vi "QueueEvent.vi"(8 "Error In":errorcluster, 9 "Event Description":string, 10 "Event Name":string, 11 "Queue In":refnum<queue>) -> (0 "Error Out":errorcluster, 3 "Queue Out":refnum<queue>)   [LabVIEW 2014]
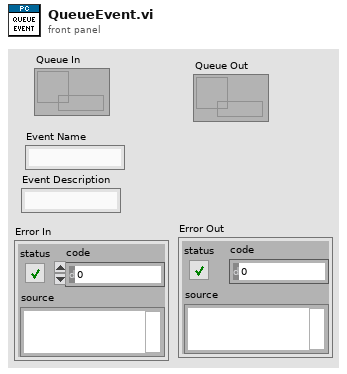
[diagram p1: front panel]
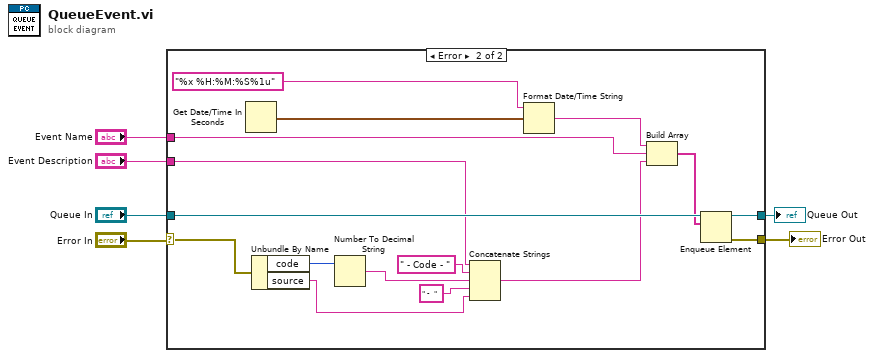
[diagram p0: block diagram]
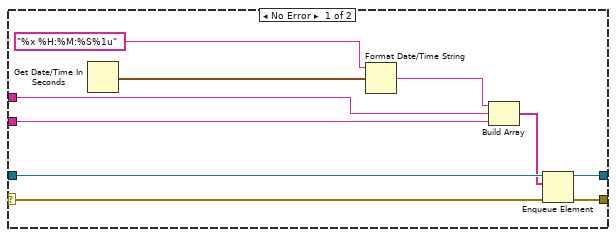
[diagram p2: hidden frame]
diagram:
  n1 = case shown="Error" "Error In" {
    selector: "Error In" -> [w11 w20]
    tunnel: [w9 w28] -> w5
    tunnel: "Queue In" -> [w10 w29]
    tunnel: "Event Name" -> [w13 w17]
    tunnel: "Event Description" -> [w12 w19]
    tunnel: [w7 w26] -> w1
    frame No Error {
      n2 = Get Date/Time In Seconds() -> (seconds since 1Jan1904=w16:timestamp)
      n3 = Format Date/Time String(time format string (%c)="%x %H:%M:%S%1u", seconds (now)=w16) -> (date/time string=w14:string)  [unwired: 1 in]
      n4 = Build Array(w14, w13, w12) -> (w8:string[])
      n5 = Enqueue Element(queue=w10, element=w8, error in (no error)=w11) -> (queue out=w7:refnum<queue>, error out=w9:errorcluster)  [unwired: 1 in, 1 out]
    }
    frame Error {
      n6 = Get Date/Time In Seconds() -> (seconds since 1Jan1904=w32:timestamp)
      n7 = Unbundle By Name(w20) -> ("code"=w25:i32, "source"=w21:string)
      n8 = Number To Decimal String(number=w25) -> (decimal integer string=w23:string)  [unwired: 1 in]
      n9 = Concatenate Strings(w19, " - Code - " ("Event Name"), w23, " -  " ("Event Name"), w21) -> (w18:string)
      n10 = Format Date/Time String(time format string (%c)="%x %H:%M:%S%1u", seconds (now)=w32) -> (date/time string=w30:string)  [unwired: 1 in]
      n11 = Build Array(w30, w17, w18) -> (w27:string[])
      n12 = Enqueue Element(queue=w29, element=w27) -> (queue out=w26:refnum<queue>, error out=w28:errorcluster)  [unwired: 2 in, 1 out]
    }
  }
  "Error Out" <- w5
  "Queue Out" <- w1
